vi "HEWH Temperature Filter.vi"(7 "Good Scan?":bool, 9 "Temperature 3 Inlet":dbl, 10 "Temperature 2 Inlet":dbl, 11 "Temperature 1 Inlet":dbl) -> (1 "Temperature 3 Outlet":dbl, 2 "Temperature 2 Outlet":dbl, 3 "Temperature 1 Outlet":dbl)   [LabVIEW 2019]
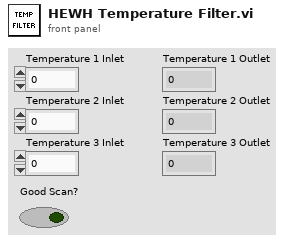
[diagram p1: front panel]
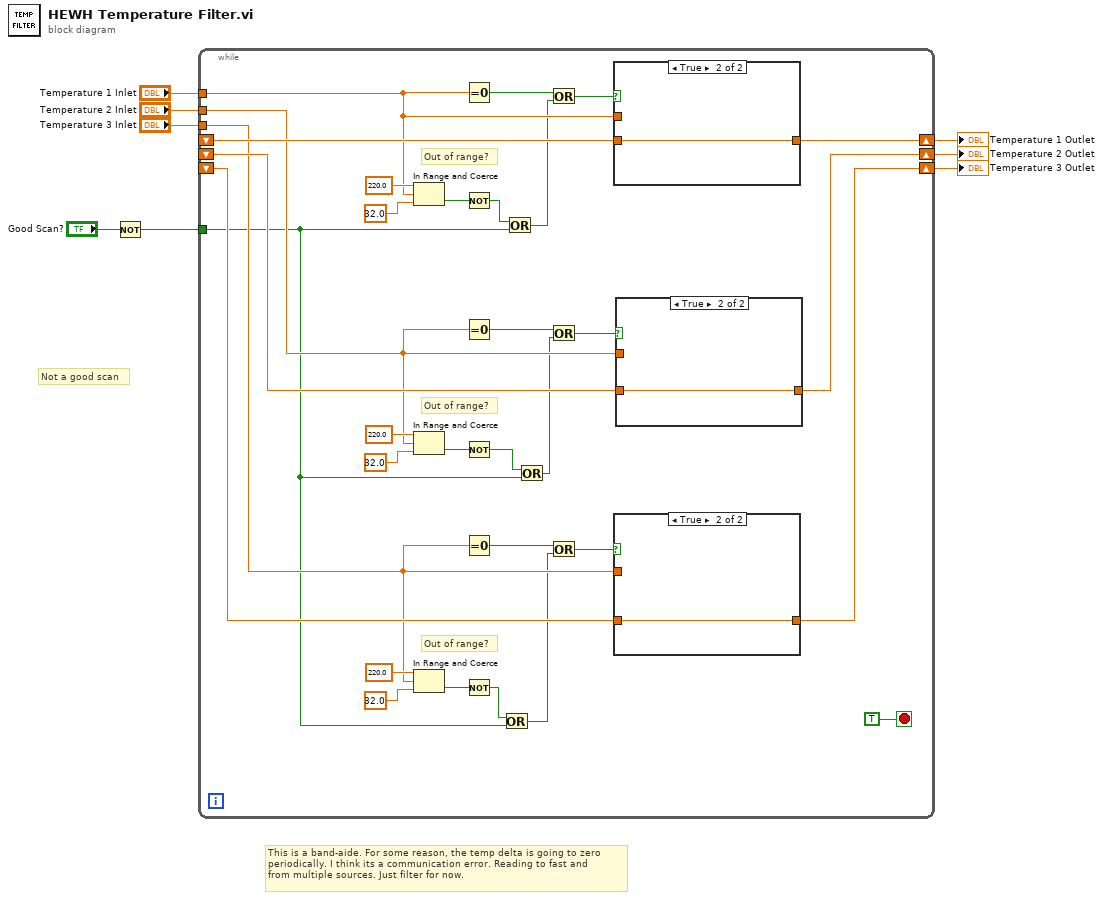
[diagram p0: block diagram]
diagram:
  # "Not a good scan"
  # "This is a band-aide. For some reason, the temp delta is going to zero\nperiodically. I think its a communication error. Reading to fast and \nfrom multiple sources. Just filter for now."
  n1 = Not(x="Good Scan?") -> (.not. x?=w1:bool)
  n2 = while {
    tunnel: "Temperature 1 Inlet" -> [w30]
    tunnel: "Temperature 2 Inlet" -> [w24]
    shift-right: [w37] -> w7
    shift-left: _ -> [w36]
    shift-right: [w39] -> w5
    shift-left: _ -> [w38]
    shift-right: [w35] -> w8
    shift-left: _ -> [w34]
    tunnel: "Temperature 3 Inlet" -> [w18]
    tunnel: w1 -> [w9]
    stop <- TRUE stop-if-true
    # "Out of range?"
    # "Out of range?"
    # "Out of range?"
    n3 = In Range and Coerce(upper limit=220.0, x=w30, lower limit=32.0) -> (In Range?=w33:bool)  [unwired: 1 out]
    n4 = In Range and Coerce(upper limit=220.0, x=w24, lower limit=32.0) -> (In Range?=w25:bool)  [unwired: 1 out]
    n5 = In Range and Coerce(upper limit=220.0, x=w18, lower limit=32.0) -> (In Range?=w21:bool)  [unwired: 1 out]
    n6 = Equal To 0?(x=w30) -> (x = 0?=w29:bool)
    n7 = Not(x=w33) -> (.not. x?=w15:bool)
    n8 = Equal To 0?(x=w24) -> (x = 0?=w23:bool)
    n9 = Not(x=w25) -> (.not. x?=w13:bool)
    n10 = Equal To 0?(x=w18) -> (x = 0?=w17:bool)
    n11 = Not(x=w21) -> (.not. x?=w11:bool)
    n12 = Or(x=w11, y=w9) -> (x .or. y?=w10:bool)
    n13 = Or(x=w15, y=w9) -> (x .or. y?=w14:bool)
    n14 = Or(x=w13, y=w9) -> (x .or. y?=w12:bool)
    n15 = Or(x=w29, y=w14) -> (x .or. y?=w28:bool)
    n16 = Or(x=w23, y=w12) -> (x .or. y?=w22:bool)
    n17 = Or(x=w17, y=w10) -> (x .or. y?=w16:bool)
    n18 = case shown="True" w28 {
      tunnel: w30 -> [w45 _]
      tunnel: [w45 w46] -> w39
      tunnel: w38 -> [_ w46]
      frame False {
      }
      frame True {
      }
    }
    n19 = case shown="True" w16 {
      tunnel: w34 -> [_ w42]
      tunnel: [w41 w42] -> w35
      tunnel: w18 -> [w41 _]
      frame False {
      }
      frame True {
      }
    }
    n20 = case shown="True" w22 {
      tunnel: w24 -> [w43 _]
      tunnel: [w43 w44] -> w37
      tunnel: w36 -> [_ w44]
      frame False {
      }
      frame True {
      }
    }
  }
  "Temperature 3 Outlet" <- w8
  "Temperature 2 Outlet" <- w7
  "Temperature 1 Outlet" <- w5
